vi "TDMS_File_Writer.vi"(11 "TDMS Cluster":T1) -> ()   [LabVIEW 2016]
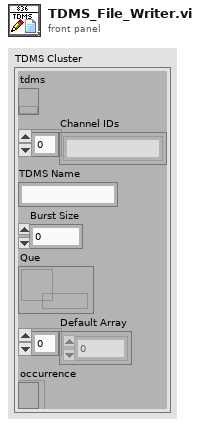
[diagram p1: front panel]
types:
  T1 = cluster{"tdms":refnum<k34>, "Channel IDs":string[], "TDMS Name":string, "Burst Size":i32, "Que":refnum<k33>, "Default Array":dbl[], "occurrence":refnum<k4>}
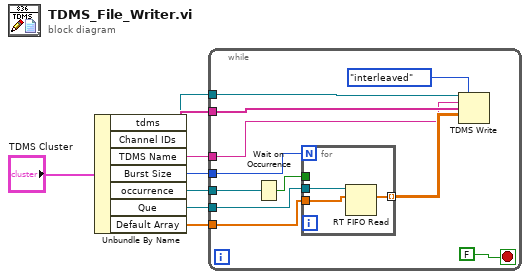
[diagram p0: block diagram]
diagram:
  n1 = Unbundle By Name("TDMS Cluster") -> ("tdms"=w1:refnum<k34>, "Channel IDs"=w2:string[], "TDMS Name"=w3:string, "Burst Size"=w4:i32, "occurrence"=w5:refnum<k4>, "Que"=w6:refnum<k33>, "Default Array"=w7:dbl[])
  n2 = while {
    tunnel: w5 -> [w10]
    tunnel: w6 -> [w18]
    tunnel: w7 -> [w17]
    tunnel: w2 -> [w15]
    tunnel: w3 -> [w14]
    tunnel: w1 -> [w12]
    tunnel: w4 -> [w11]
    stop <- FALSE stop-if-true
    n3 = Wait on Occurrence(2:w10) -> (0:w9:bool)  [unwired: 2 in]
    n4 = for {
      N: w11 -> [_]
      tunnel: w18 -> [w22]
      tunnel: w17 -> [w21]
      tunnel: [w20] -> w16 mode=indexing
      tunnel: w9 -> [_]
      n5 = RT FIFO Read(0:w22, 1:w21) -> (9:w20:dbl[])  [unwired: 2 in, 4 out]
    }
    n6 = TDMS Write(0:w12, 1:enum16{"decimated", "interleaved"}."interleaved" ("data layout (0:decimated)"), 5:w14, 7:w15, 9:w16) -> ()  [unwired: 1 in, 4 out]
  }
